vi "DeleteRegistry - Shell Menu.vi"   [LabVIEW 2017]
uses:
  <vilib>/registry/registry.llb/Registry RtKey.ctl
types:
  T1 = enum32{"Invalid", "Standard", "Closed", "Hidden", "Minimized", "Maximized"}
  T2 = typedef "Registry RtKey.ctl" = enum32{"HKEY_CLASSES_ROOT", "HKEY_CURRENT_USER", "HKEY_LOCAL_MACHINE", "HKEY_USERS", "HKEY_PERFORMANCE_DATA", "HKEY_CURRENT_CONFIG", "HKEY_DYN_DATA"}
  T3 = typedef "Registry refnum.ctl" = refnum<k1>
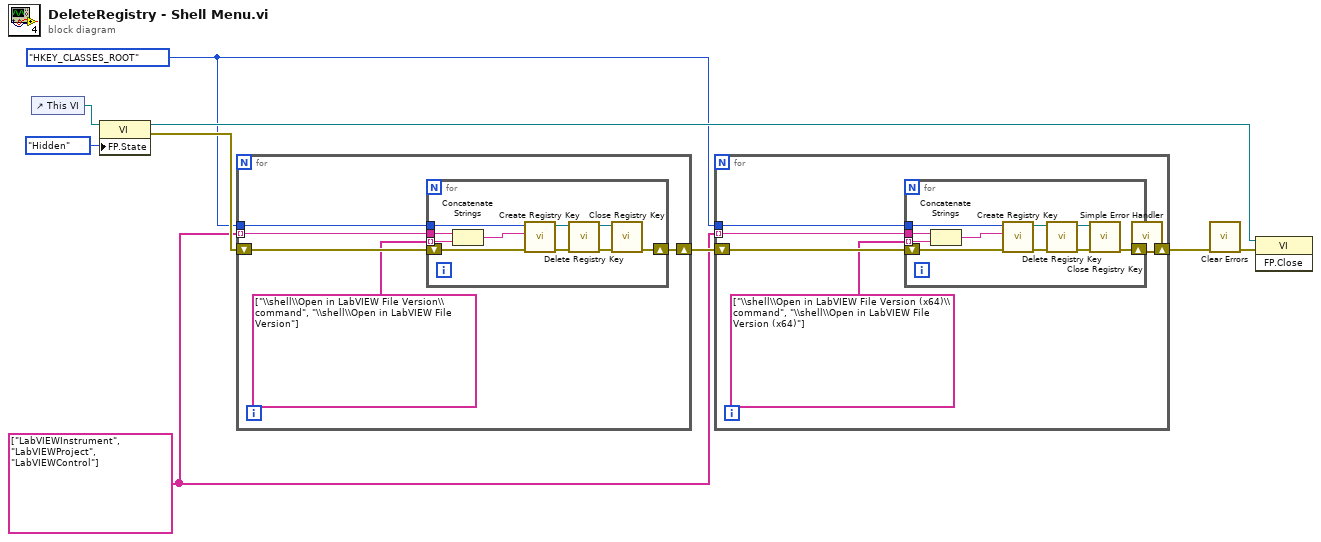
[diagram p0: block diagram]
diagram:
  w1 = string[] ["LabVIEWInstrument", "LabVIEWProject", "LabVIEWControl"]
  w2 = Registry_RtKey."HKEY_CLASSES_ROOT" ("root key (HKEY_LOCAL_MACHINE)")
  n1 = control-ref of="This VI"() -> (w9:refnum<vi>)
  n2 = property class="VI"(reference=w9, "FP.State"=T1."Hidden" ("Front Panel Window:State")) -> (reference out=w5:refnum<vi>, error out=w4:errorcluster)  [unwired: 1 in]
  n3 = for {
    tunnel: w2 -> [w14]
    tunnel: w1 -> [w13] mode=indexing
    shift-right: [w12] -> w3
    shift-left: w4 -> [w11]
    n4 = for {
      tunnel: w14 -> [w20]
      tunnel: w13 -> [w18]
      shift-right: [w17] -> w12
      shift-left: w11 -> [w16]
      tunnel: string[] ["\\shell\\Open in LabVIEW File Version\\command", "\\shell\\Open in LabVIEW File Version"] -> [w15] mode=indexing
      n5 = Concatenate Strings(w18, w15) -> (w19:string)
      n6 = call <vilib>:"Create Registry Key.vi"("error in (no error)"=w16, "subkey"=w19, "root key (HKEY_LOCAL_MACHINE)"=w20) -> ("error out"=w23:errorcluster, "refnum out"=w24:T3)  [unwired: 6 in, 1 out]
      n7 = call <vilib>:"Delete Registry Key.vi"("error in (no error)"=w23, "refnum"=w24) -> ("error out"=w21:errorcluster, "refnum out"=w22:T3)  [unwired: 8 in]
      n8 = call <vilib>:"Close Registry Key.vi"("error in (no error)"=w21, "refnum"=w22) -> ("error out"=w17:errorcluster)  [unwired: 5 in]
    }
  }
  n9 = for {
    tunnel: w2 -> [w29]
    tunnel: w1 -> [w28] mode=indexing
    shift-right: [w27] -> _
    shift-left: w3 -> [w26]
    n10 = for {
      tunnel: w29 -> [w35]
      tunnel: w28 -> [w33]
      shift-right: [w32] -> w27
      shift-left: w26 -> [w31]
      tunnel: string[] ["\\shell\\Open in LabVIEW File Version (x64)\\command", "\\shell\\Open in LabVIEW File Version (x64)"] -> [w30] mode=indexing
      n11 = Concatenate Strings(w33, w30) -> (w34:string)
      n12 = call <vilib>:"Create Registry Key.vi"("error in (no error)"=w31, "subkey"=w34, "root key (HKEY_LOCAL_MACHINE)"=w35) -> ("error out"=w38:errorcluster, "refnum out"=w39:T3)  [unwired: 6 in, 1 out]
      n13 = call <vilib>:"Delete Registry Key.vi"("error in (no error)"=w38, "refnum"=w39) -> ("error out"=w36:errorcluster, "refnum out"=w37:T3)  [unwired: 8 in]
      n14 = call <vilib>:"Close Registry Key.vi"("error in (no error)"=w36, "refnum"=w37) -> ("error out"=w32:errorcluster)  [unwired: 5 in]
    }
  }
  n15 = call <vilib>:"Simple Error Handler.vi"("error in (no error)"=w3) -> ("error out"=w7:errorcluster)  [unwired: 4 in, 4 out]
  n16 = call <vilib>:"Clear Errors.vi"("error in (no error)"=w7) -> ("error out"=w6:errorcluster)  [unwired: 5 in, 1 out]
  n17 = invoke class="VI" method="FP.Close"(reference=w5, error in=w6) -> ()  [unwired: 1 in, 3 out]
